vi "Auto Command Parsing.vi"(10 "Command Paremeters":dbl, 11 "Command code In":string) -> (2 "Abort":bool, 3 "No Command?":bool)   [LabVIEW 2017]
uses:
  Robot Global Data.vi
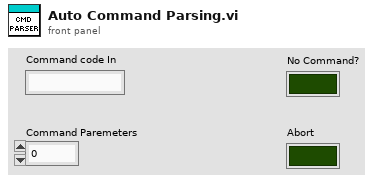
[diagram p1: front panel]
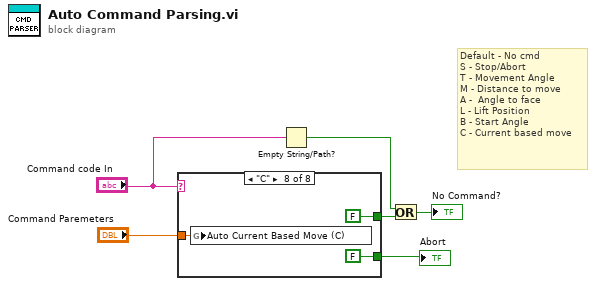
[diagram p0: block diagram]
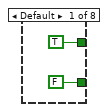
[diagram p2: hidden frame]
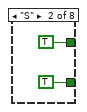
[diagram p3: hidden frame]
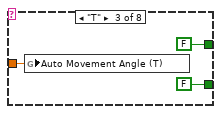
[diagram p4: hidden frame]
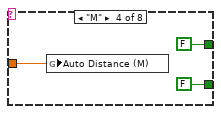
[diagram p5: hidden frame]
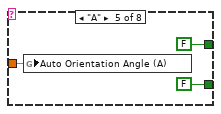
[diagram p6: hidden frame]
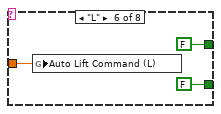
[diagram p7: hidden frame]
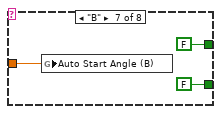
[diagram p8: hidden frame]
diagram:
  # "Default - No cmd\nS - Stop/Abort\nT - Movement Angle\nM - Distance to move\nA -  Angle to face\nL - Lift Position\nB - Start Angle\nC - Current based move"
  n1 = case shown="\"C\"" "Command code In" {
    tunnel: [TRUE TRUE FALSE FALSE FALSE FALSE FALSE FALSE] -> w6
    tunnel: [FALSE TRUE FALSE FALSE FALSE FALSE FALSE FALSE] -> w5
    tunnel: "Command Paremeters" -> [_ _ w11 w14 w17 w20 w23 w26]
    frame Default {
    }
    frame "S" {
    }
    frame "T" {
      n2 = global write "Robot Global Data.vi" "Auto Movement Angle (T)"(w11) -> ()
    }
    frame "M" {
      n3 = global write "Robot Global Data.vi" "Auto Distance (M)"(w14) -> ()
    }
    frame "A" {
      n4 = global write "Robot Global Data.vi" "Auto Orientation Angle (A)"(w17) -> ()
    }
    frame "L" {
      n5 = global write "Robot Global Data.vi" "Auto Lift Command (L)"(w20) -> ()
    }
    frame "B" {
      n6 = global write "Robot Global Data.vi" "Auto Start Angle (B)"(w23) -> ()
    }
    frame "C" {
      n7 = global write "Robot Global Data.vi" "Auto Current Based Move (C)"(w26) -> ()
    }
  }
  "Abort" <- w5
  n8 = Empty String/Path?(string/path="Command code In") -> (empty?=w1:bool)
  n9 = Or(x=w1, y=w6) -> (x .or. y?=→"No Command?":bool)
